vi "fit from queues.vi"(5 "redo initial guess (T)":bool=TRUE, 6 "min mag streangth (T mm^3)":dbl=100.0 format="%#_13g", 7 "max mag streangth (T mm^3)":dbl=1000.0 format="%#_13g", 8 "error in (no error)":errorcluster, 10 "max number to fit":u16=100, 11 "display queues":T1) -> (0 "error out":errorcluster)   [LabVIEW 2017]
uses:
  typedefs/queue cluster.ctl
  typedefs/reading queue.ctl
  typedefs/reading.ctl
  typedefs/readingType.ctl
  typedefs/magnetomter reading set.ctl
  typedefs/magnet location with timestamp.ctl
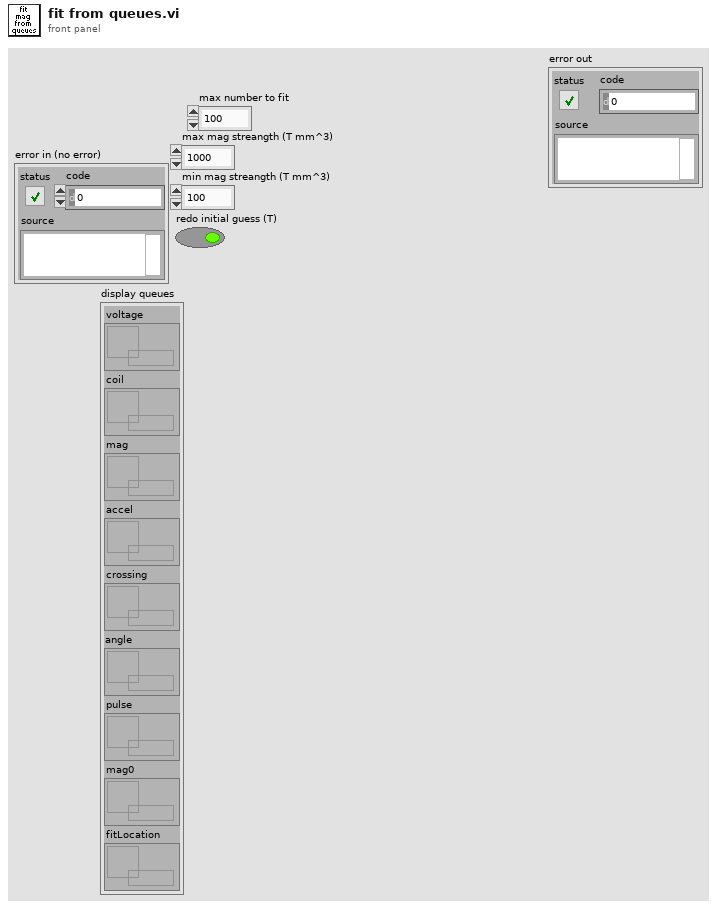
[diagram p1: front panel]
types:
  T1 = typedef "queue cluster.ctl" = cluster{"voltage":T2, "coil":T2, "mag":refnum<queue>, "accel":T2, "crossing":T2, "angle":T2, "pulse":T2, "mag0":T2, "fitLocation":refnum<queue>}
  T2 = typedef "reading queue.ctl" = refnum<queue>
  T3 = typedef "magnetomter reading set.ctl" = cluster{"time":fxp<+,48,48>, "mag readings":cluster{"magnetometer index":dbl, "Bx":dbl, "By":dbl, "Bz":dbl, "magnetometer x":dbl, "magnetometer y":dbl}[]}
  T4 = typedef "magnet location with timestamp.ctl" = cluster{"x magnet":dbl, "y magnet":dbl, "z magnet":dbl, "Br*V (T*mm^3)":dbl, "theta - moment angle to z-axis":dbl, "phi - moment angle to x-axis":dbl, "measurement time":dbl}
  T5 = typedef "magnet location fit result.ctl" = cluster{"x magnet":dbl, "y magnet":dbl, "z magnet":dbl, "Br*V (T*mm^3)":dbl, "theta - moment angle to z-axis":dbl, "phi - moment angle to x-axis":dbl}
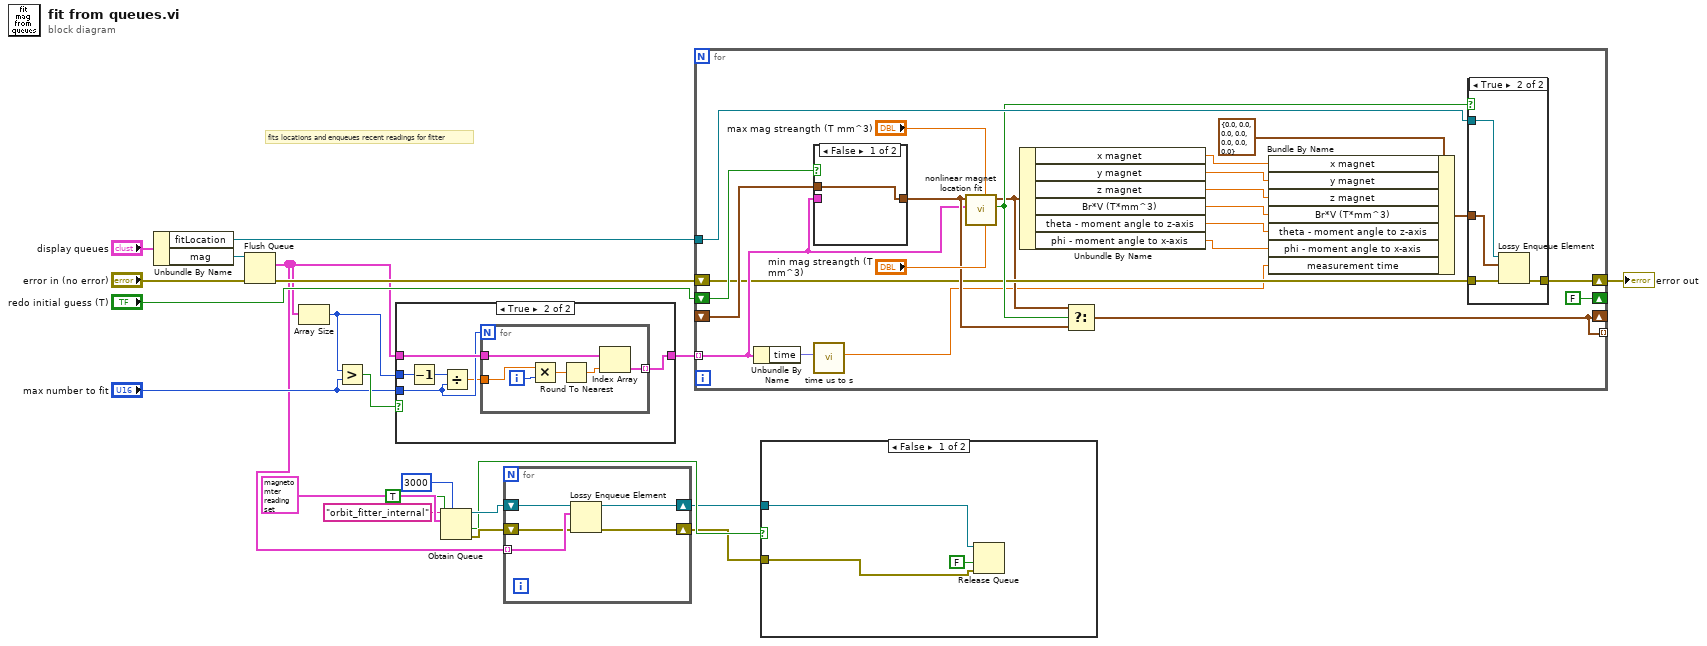
[diagram p0: block diagram]
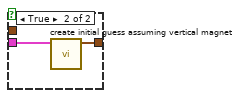
[diagram p4: hidden frame]
diagram:
  # "fits locations and enqueues recent readings for fitter"
  n1 = Unbundle By Name("display queues") -> ("fitLocation"=w13:refnum<queue>, "mag"=w12:refnum<queue>)
  n2 = Flush Queue(queue=w12, error in (no error)="error in (no error)") -> (remaining elements=w1:T3[], error out=w15:errorcluster)  [unwired: 1 out]
  n3 = Array Size(array=w1) -> (size(s)=w19:i32)
  n4 = Greater?(x=w19, y="max number to fit") -> (0:w20:bool)
  n5 = case shown="True" w20 {
    tunnel: w1 -> [w22 w27]
    tunnel: w19 -> [_ w28]
    tunnel: "max number to fit" -> [_ w26]
    tunnel: [w22 w23] -> w17
    frame False {
    }
    frame True {
      n6 = Decrement(x=w28) -> (x-1=w24:i32)
      n7 = Divide(x=w24, y=w26) -> (x/y=w25:dbl)
      n8 = for {
        N: w26 -> [_]
        tunnel: w27 -> [w31]
        tunnel: w25 -> [w33]
        tunnel: [w29] -> w23 mode=indexing
        i -> [w34]
        n9 = Multiply(x=w33, y=w34) -> (x*y=w32:dbl)
        n10 = Round To Nearest(number=w32) -> (nearest integer value=w30:dbl)
        n11 = Index Array(array=w31, index=w30) -> (element=w29:T3)
      }
    }
  }
  n12 = Obtain Queue(max queue size (-1, unlimited)=3000, name (unnamed)="orbit_fitter_internal", element data type=T3 {"time"=0.0, "mag readings"=[]} ("Magnetometer reading set"), create if not found? (T)=TRUE) -> (queue out=w6:refnum<queue>, created new?=w4:bool, error out=w5:errorcluster)  [unwired: 1 in]
  n13 = for {
    tunnel: w1 -> [w38] mode=indexing
    shift-right: [w36] -> w3
    shift-left: w5 -> [w37]
    shift-right: [w35] -> w2
    shift-left: w6 -> [w39]
    n14 = Lossy Enqueue Element(queue=w39, element=w38, error in (no error)=w37) -> (queue out=w35:refnum<queue>, error out=w36:errorcluster)  [unwired: 2 out]
  }
  n15 = for {
    tunnel: [w60] -> _ mode=indexing
    shift-right: [w60] -> _
    shift-left: _ -> [w57]
    tunnel: w17 -> [w54] mode=indexing
    shift-right: [FALSE ("redo initial guess")] -> _
    shift-left: "redo initial guess (T)" -> [w59]
    tunnel: w13 -> [w55]
    shift-right: [w51] -> w11
    shift-left: w15 -> [w52]
    n16 = Unbundle By Name(w54) -> ("time"=w42:fxp<+,48,48>)
    n17 = case shown="False" w59 {
      tunnel: w54 -> [_ w70]
      tunnel: w57 -> [w68 _]
      tunnel: [w68 w69] -> w56
      frame False {
      }
      frame True {
        n18 = call "create initial guess assuming vertical magnet.vi"("Magnetometer reading set"=w70) -> ("initial guess"=w69:T5)  [unwired: 10 in]
      }
    }
    n19 = call "time us to s.vi"("time (us)"=w42) -> ("time (s)"=w41:dbl)  [unwired: 10 in]
    n20 = call "nonlinear magnet location fit.vi"("min mag streangth (T mm^3)"="min mag streangth (T mm^3)", "max mag streangth (T mm^3)"="max mag streangth (T mm^3)", "Magnetometer reading set"=w54, "initial parameters"=w56) -> ("fit OK"=w53:bool, "fit parameters"=w50:T5)  [unwired: 5 in, 1 out]
    n21 = Unbundle By Name(w50) -> ("x magnet"=w48:dbl, "y magnet"=w47:dbl, "z magnet"=w46:dbl, "Br*V (T*mm^3)"=w45:dbl, "theta - moment angle to z-axis"=w44:dbl, "phi - moment angle to x-axis"=w43:dbl)
    n22 = Select(t=w50, s=w53, f=w56) -> (s? t:f=w60:T5)
    n23 = Bundle By Name(cluster=T4 {"x magnet"=0.0, "y magnet"=0.0, "z magnet"=0.0, "Br*V (T*mm^3)"=0.0, "theta - moment angle to z-axis"=0.0, "phi - moment angle to x-axis"=0.0, "measurement time"=0.0} ("element"), "x magnet"=w48, "y magnet"=w47, "z magnet"=w46, "Br*V (T*mm^3)"=w45, "theta - moment angle to z-axis"=w44, "phi - moment angle to x-axis"=w43, "measurement time"=w41) -> (w40:T4)
    n24 = case shown="True" w53 {
      tunnel: w55 -> [_ w67]
      tunnel: w52 -> [w63 w66]
      tunnel: [w63 w65] -> w51
      tunnel: w40 -> [_ w64]
      frame False {
      }
      frame True {
        n25 = Lossy Enqueue Element(queue=w67, element=w64, error in (no error)=w66) -> (error out=w65:errorcluster)  [unwired: 3 out]
      }
    }
  }
  "error out" <- w11
  n26 = case shown="False" w4 {
    tunnel: w3 -> [w71 _]
    tunnel: w2 -> [w73 _]
    frame False {
      n27 = Release Queue(queue=w73, force destroy? (F)=FALSE, error in (no error)=w71) -> ()  [unwired: 3 out]
    }
    frame True {
    }
  }
